vi "Untitled 4.vi"() -> ()   [LabVIEW 2014, in "TableLogger_Actor.lvlib" / "TableLogger_Actor.lvclass"]
uses:
  TableLogger_Actor.lvclass
  <userlib>/_OpenG.lib/array/array.llb/Filter 1D Array with Scalar (String)__ogtk.vi
  <vilib>/Utility/file.llb/Read From Spreadsheet File (string).vi
panel:
  out "all rows":string[][](array[string])=[["Numeric Data", "Float Data", "String Data", "Enum Data", "Array Data 2[0].Numeric Data", "Array Data 2[1].Numeric Data", "Array Data 2[2].Numeric Data", "Cluster 2.String", "Cluster 2.Array Data 2[0].Numeric Data", "Cluster 2.Array Data 2[1].Numeric Data", "Cluster 2.Array Data 2[2].Numeric Data", "Cluster 3.Cluster78.Array Data 2[0].Numeric Data", "Cluster 3.Cluster78.Array Data 2[1].Numeric Data", "Cluster 3.Cluster78.Array Data 2[2].Numeric Data", "Enum Data 2", "String Data 2", "Float Data 2", "Array Data[0].Numeric Data", "Array Data[1].Numeric Data", "Array Data[2].Numeric Data", "Array Data[3].Numeric Data", "Array A[0].Cluster A.String A", "Array A[0].Cluster A.Array B[0].Cluster B.String B", "Array A[0].Cluster A.Array B[0].Cluster B.Array B 2[0].Cluster B.String B", "Array A[0].Cluster A.Array B[0].Cluster B.Array B 2[1].Cluster B.String B", "Array A[0].Cluster A.Array B[0].Cluster B.Array B 2[2].Cluster B.String B", "Array A[0].Cluster A.Array B[1].Cluster B.String B", "Array A[0].Cluster A.Array B[1].Cluster B.Array B 2[0].Cluster B.String B", "Array A[0].Cluster A.Array B[1].Cluster B.Array B 2[1].Cluster B.String B", "Array A[0].Cluster A.Array B[1].Cluster B.Array B 2[2].Cluster B.String B", "Array A[0].Cluster A.Array B[2].Cluster B.String B", "Array A[0].Cluster A.Array B[2].Cluster B.Array B 2[0].Cluster B.String B", "Array A[0].Cluster A.Array B[2].Cluster B.Array B 2[1].Cluster B.String B", "Array A[0].Cluster A.Array B[2].Cluster B.Array B 2[2].Cluster B.String B", "Array A[0].Cluster A.Array B 2[0].Cluster B.String B", "Array A[0].Cluster A.Array B 2[1].Cluster B.String B", "Array A[0].Cluster A.Array B 2[2].Cluster B.String B", "Array A[1].Cluster A.String A", "Array A[1].Cluster A.Array B[0].Cluster B.String B", "Array A[1].Cluster A.Array B[0].Cluster B.Array B 2[0].Cluster B.String B", "Array A[1].Cluster A.Array B[0].Cluster B.Array B 2[1].Cluster B.String B", "Array A[1].Cluster A.Array B[0].Cluster B.Array B 2[2].Cluster B.String B", "Array A[1].Cluster A.Array B[1].Cluster B.String B", "Array A[1].Cluster A.Array B[1].Cluster B.Array B 2[0].Cluster B.String B", "Array A[1].Cluster A.Array B[1].Cluster B.Array B 2[1].Cluster B.String B", "Array A[1].Cluster A.Array B[1].Cluster B.Array B 2[2].Cluster B.String B", "Array A[1].Cluster A.Array B[2].Cluster B.String B", "Array A[1].Cluster A.Array B[2].Cluster B.Array B 2[0].Cluster B.String B", "Array A[1].Cluster A.Array B[2].Cluster B.Array B 2[1].Cluster B.String B", "Array A[1].Cluster A.Array B[2].Cluster B.Array B 2[2].Cluster B.String B", "Array A[1].Cluster A.Array B 2[0].Cluster B.String B", "Array A[1].Cluster A.Array B 2[1].Cluster B.String B", "Array A[1].Cluster A.Array B 2[2].Cluster B.String B"], ["0", "0.0", "", "Enum Item 1", "0", "0", "0", "", "0", "0", "0", "0", "0", "0", "Enum Item 1", "", "0.0", "0", "0", "0", "4", "hello", "uq", "u", "c", "hello", "c", "u", "c", "hello", "hello", "u", "c", "hello", "u", "c", "hello", "hello", "uP", "u", "c", "hello", "c", "u", "c", "hello", "hello", "u", "c", "hello", "u", "c", "hello"], ["401", "0.0", "q", "Enum Item 1", "0", "0", "0", "", "0", "0", "0", "0", "0", "0", "Enum Item 1", "", "0.0", "0", "0", "0", "4", "hello", "uq", "u", "c", "hello", "c", "u", "c", "hello", "hello", "u", "c", "hello", "u", "c", "hello", "hello", "uP", "u", "c", "hello", "c", "u", "c", "hello", "hello", "u", "c", "hello", "u", "c", "hello"], ["0", "0.0", "", "Enum Item 1", "0", "0", "0", "", "0", "0", "0", "0", "0", "0", "Enum Item 1", "", "0.0", "0", "0", "0", "4", "hello", "uq", "u", "c", "hello", "c", "u", "c", "hello", "hello", "u", "c", "hello", "u", "c", "hello", "hello", "uP", "u", "c", "hello", "c", "u", "c", "hello", "hello", "u", "c", "hello", "u", "c", "hello"], ["0", "0.0", "", "Enum Item 1", "0", "0", "0", "", "0", "0", "0", "0", "0", "0", "Enum Item 1", "", "0.0", "0", "0", "0", "4", "hello", "uq", "u", "c", "hello", "c", "u", "c", "hello", "hello", "u", "c", "hello", "u", "c", "hello", "hello", "uP", "u", "c", "hello", "c", "u", "c", "hello", "hello", "u", "c", "hello", "u", "c", "hello"], ["0", "0.0", "", "Enum Item 1", "0", "0", "0", "", "0", "0", "0", "0", "0", "0", "Enum Item 1", "", "0.0", "0", "0", "0", "4", "hello", "uq", "u", "c", "hello", "c", "u", "c", "hello", "hello", "u", "c", "hello", "u", "c", "hello", "hello", "uP", "u", "c", "hello", "c", "u", "c", "hello", "hello", "u", "c", "hello", "u", "c", "hello"], ["0", "0.0", "", "Enum Item 1", "0", "0", "0", "", "0", "0", "0", "0", "0", "0", "Enum Item 1", "", "0.0", "0", "0", "0", "4", "hello", "uq", "u", "c", "hello", "c", "u", "c", "hello", "hello", "u", "c", "hello", "u", "c", "hello", "hello", "uP", "u", "c", "hello", "c", "u", "c", "hello", "hello", "u", "c", "hello", "u", "c", "hello"], ["0", "0.0", "", "Enum Item 1", "0", "0", "0", "", "0", "0", "0", "0", "0", "0", "Enum Item 1", "", "0.0", "0", "0", "0", "4", "hello", "uq", "u", "c", "hello", "c", "u", "c", "hello", "hello", "u", "c", "hello", "u", "c", "hello", "hello", "uP", "u", "c", "hello", "c", "u", "c", "hello", "hello", "u", "c", "hello", "u", "c", "hello"], ["0", "0.0", "", "Enum Item 1", "0", "0", "0", "", "0", "0", "0", "0", "0", "0", "Enum Item 1", "", "0.0", "0", "0", "0", "4", "hello", "uq", "u", "c", "hello", "c", "u", "c", "hello", "hello", "u", "c", "hello", "u", "c", "hello", "hello", "uP", "u", "c", "hello", "c", "u", "c", "hello", "hello", "u", "c", "hello", "u", "c", "hello"], ["0", "0.0", "", "Enum Item 1", "0", "0", "0", "", "0", "0", "0", "0", "0", "0", "Enum Item 1", "", "0.0", "0", "0", "0", "4", "hello", "uq", "u", "c", "hello", "c", "u", "c", "hello", "hello", "u", "c", "hello", "u", "c", "hello", "hello", "uP", "u", "c", "hello", "c", "u", "c", "hello", "hello", "u", "c", "hello", "u", "c", "hello"], ["0", "0.0", "", "Enum Item 1", "0", "0", "0", "", "0", "0", "0", "0", "0", "0", "Enum Item 1", "", "0.0", "0", "0", "0", "4", "hello", "uq", "u", "c", "hello", "c", "u", "c", "hello", "hello", "u", "c", "hello", "u", "c", "hello", "hello", "uP", "u", "c", "hello", "c", "u", "c", "hello", "hello", "u", "c", "hello", "u", "c", "hello"], ["0", "0.0", "", "Enum Item 1", "0", "0", "0", "", "0", "0", "0", "0", "0", "0", "Enum Item 1", "", "0.0", "0", "0", "0", "4", "hello", "uq", "u", "c", "hello", "c", "u", "c", "hello", "hello", "u", "c", "hello", "u", "c", "hello", "hello", "uP", "u", "c", "hello", "c", "u", "c", "hello", "hello", "u", "c", "hello", "u", "c", "hello"], ["401", "0.0", "", "Enum Item 1", "0", "0", "0", "", "0", "0", "0", "0", "0", "0", "Enum Item 1", "", "0.0", "0", "0", "0", "4", "hello", "uq", "u", "c", "hello", "c", "u", "c", "hello", "hello", "u", "c", "hello", "u", "c", "hello", "hello", "uP", "u", "c", "hello", "c", "u", "c", "hello", "hello", "u", "c", "hello", "u", "c", "hello"]]
  in  "LV Data":T1={"Numeric Data"=0, "Float Data"=0.0, "String Data"="", "Enum Data"=enum."Enum Item 1", "Array Data 2"=[0, 0, 7], "Cluster 2"={"String"="", "Array Data 2"=[0, 0, 8]}, "Cluster 3"={"Cluster78"={"Array Data 2"=[0, 0, 7]}}, "Enum Data 2"=enum."Enum Item 1", "String Data 2"="", "Float Data 2"=0.0, "Array Data"=[0, 9], "Array A"=[{"String A"="hello", "Array B"=[{"String B"="u", "Array B 2"=[]}, {"String B"="c", "Array B 2"=[]}, {"String B"="hello", "Array B 2"=[]}], "Array B 2"=[{"String B"="u"}, {"String B"="c"}, {"String B"="hello"}]}, {"String A"="hello", "Array B"=[{"String B"="u", "Array B 2"=[]}, {"String B"="c", "Array B 2"=[]}, {"String B"="hello", "Array B 2"=[]}], "Array B 2"=[{"String B"="up"}, {"String B"="c"}, {"String B"="hello"}]}]}
  out "Headers 4":string[](array[string])
  out "offset of match":i32
  out "number of replacements":i32
  in  "String":string
  out "Indices of Elements":i32[](array[numeric])
  in  "Array":string[](array[string])
  out "output 4":string
  out "output 3":i32
  out "Headers 3":string[](array[string])
  out "Headers 2":string[](array[string])
  in  "Cluster 2":cluster{"Array":i32[], "Numeric":i32}
  in  "Cluster":cluster{"Array":i32[], "Numeric":i32}
  out "remaining string":string
  out "output 2":string
  out "output 1":string
  in  "HeaderPrefix":string
  out "output string":string
  out "selection":bool
  in  "string":string
  out "Headers":string[](array[string])
  in  "ClusterA":T2
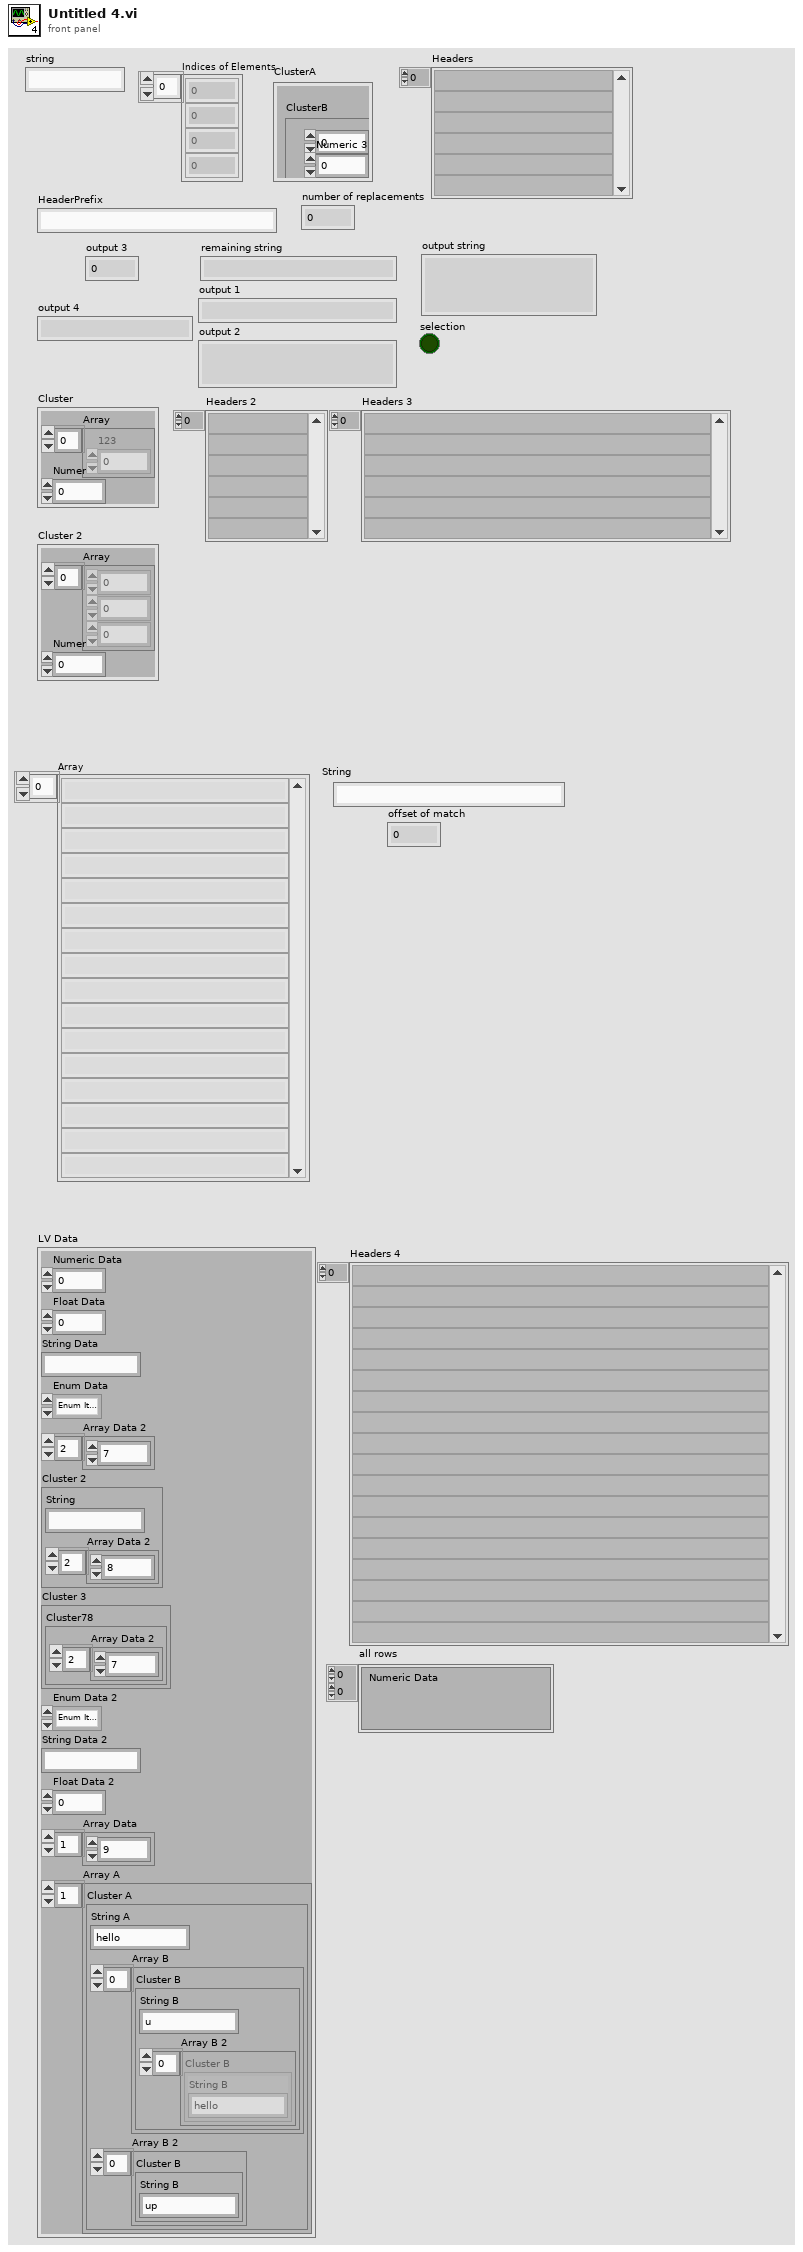
[diagram p1: front panel]
types:
  T1 = cluster{"Numeric Data":i32, "Float Data":dbl, "String Data":string, "Enum Data":enum16{"Enum Item 1", "Enum Item 2"}, "Array Data 2":i32[], "Cluster 2":cluster{"String":string, "Array Data 2":i32[]}, "Cluster 3":cluster{"Cluster78":cluster{"Array Data 2":i32[]}}, "Enum Data 2":enum16{"Enum Item 1", "Enum Item 2"}, "String Data 2":string, "Float Data 2":dbl, "Array Data":i32[], "Array A":cluster{"String A":string, "Array B":cluster{"String B":string, "Array B 2":cluster{"String B":string}[]}[], "Array B 2":cluster{"String B":string}[]}[]}
  T2 = cluster{"ClusterB":cluster{"Numeric":dbl, "Numeric 2":dbl, "Numeric 3":dbl}}
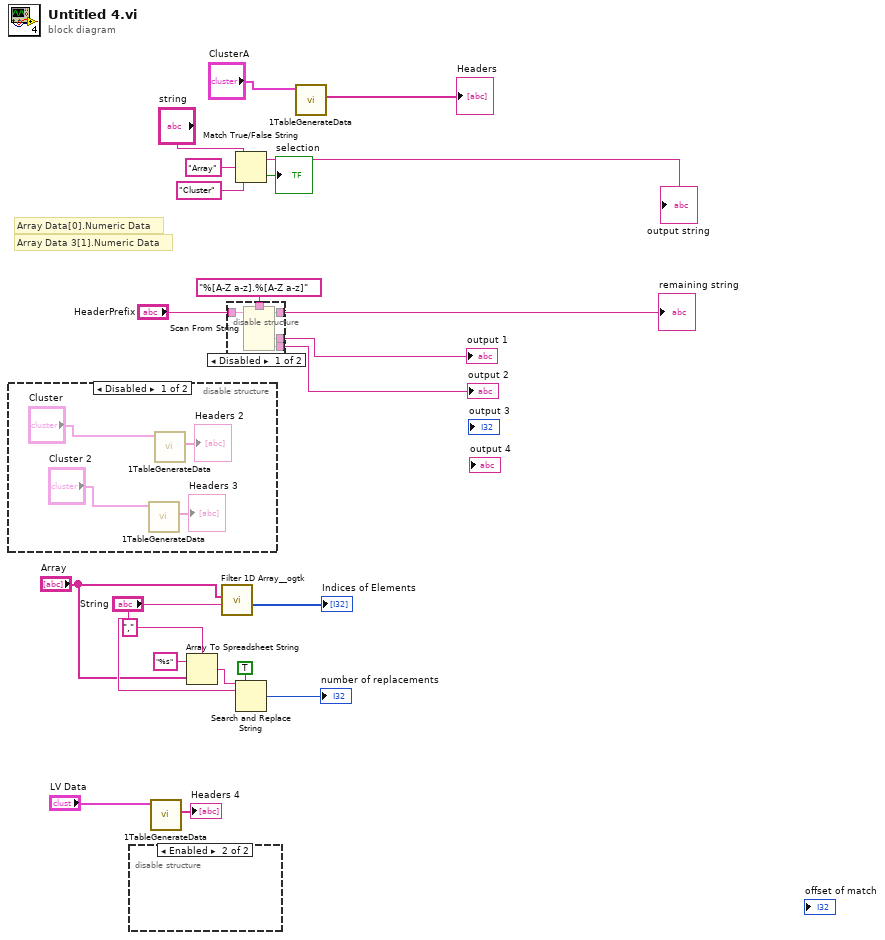
[diagram p0: block diagram]
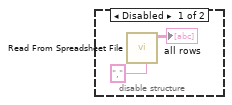
[diagram p2: hidden frame]
diagram:
  # "Array Data 3[1].Numeric Data"
  # "Array Data[0].Numeric Data"
  n1 = disable-structure shown="Disabled" {
    frame Disabled {
      n2 = call "1TableGenerateData.vi"("Cluster Variant"="Cluster 2") -> ("Headers"=→"Headers 3":string[])  [unwired: 6 in, 4 out]
      n3 = call "1TableGenerateData.vi"("Cluster Variant"="Cluster") -> ("Headers"=→"Headers 2":string[])  [unwired: 6 in, 4 out]
    }
    frame Enabled {
    }
  }
  n4 = disable-structure shown="Enabled" {
    frame Disabled {
      n5 = call-poly <vilib>:"Read From Spreadsheet File.vi"("delimiter (\\t)"="," ("delimiter (\\t)")) -> ("all rows"=→"all rows":string[][])  [unwired: 6 in, 4 out]
    }
    frame Enabled {
    }
  }
  n6 = call "1TableGenerateData.vi"("Cluster Variant"="LV Data") -> ("Headers"=→"Headers 4":string[])  [unwired: 6 in, 4 out]
  n7 = Array To Spreadsheet String(delimiter (Tab)=",", array="Array", 3:"%s" ("format string")) -> (spreadsheet string=w9:string)
  n8 = call-poly <userlib>:"Filter 1D Array__ogtk.vi"("items to filter"="String", "array"="Array") -> ("filtered item indices"=→"Indices of Elements":i32[])  [unwired: 4 in, 1 out]
  n9 = disable-structure shown="Disabled" {
    disable-tunnel: "%[A-Z a-z].%[A-Z a-z]" ("format string") -> [w33 _]
    disable-tunnel: "HeaderPrefix" -> [w32 _]
    disable-tunnel: [w31 _] -> w13
    disable-tunnel: [w30 _] -> w12
    disable-tunnel: [w29 _] -> w11
    frame Disabled {
      n10 = Scan From String(format string=w33, input string=w32) -> (remaining string=w30:string, output 1=w31:dbl, output 2=w29:dbl)  [unwired: 4 in, 2 out]
    }
    frame Enabled {
    }
  }
  "output 1" <- w13
  "output 2" <- w11
  "remaining string" <- w12
  n11 = Match True/False String(2:"Cluster" ("false string"), 3:"Array" ("true string"), 4:"string") -> (0:→"selection":bool, 1:→"output string":string)
  n12 = Search and Replace String(replace all?=TRUE ("replace all? (F)"), input string=w9, search string="String") -> (number of replacements=→"number of replacements":i32)  [unwired: 5 in, 3 out]
  n13 = call "1TableGenerateData.vi"("Cluster Variant"="ClusterA") -> ("Headers"=→"Headers":string[])  [unwired: 6 in, 4 out]
